vi "xy_graph_zoom.vi"() -> ()   [LabVIEW 2009]
uses:
  <vilib>/Utility/file.llb/Write To Spreadsheet File (DBL).vi
panel:
  out "sub-array for csv file":dbl[][](array[numeric])
  in  "stop":bool
  out "csv":bool
  out "print":bool
  in  "csv":bool
  in  "print":bool
  out "y-axis of sub-array":dbl[](array[numeric])
  out "x-axis of sub-array":dbl[](array[numeric])
  out "Y-max":dbl
  out "Y-min":dbl
  out "X-max":dbl
  out "X-min":dbl
  in  "y-axis array":dbl[](array[numeric])=[6.0, 2.0, 3.0, 9.0, 8.0, 5.0, 12.0, 14.0, 7.0, 18.0, 16.0]
  in  "x-axis array":dbl[](array[numeric])=[0.0, 2.0, 4.0, 6.0, 8.0, 10.0, 12.0, 14.0, 16.0, 18.0, 20.0]
  out "XY Graph":cluster{"Array":dbl[], "Array 2":dbl[]}(graph)
  # "these will write to C:\\temp\\ (the directory must exist)"
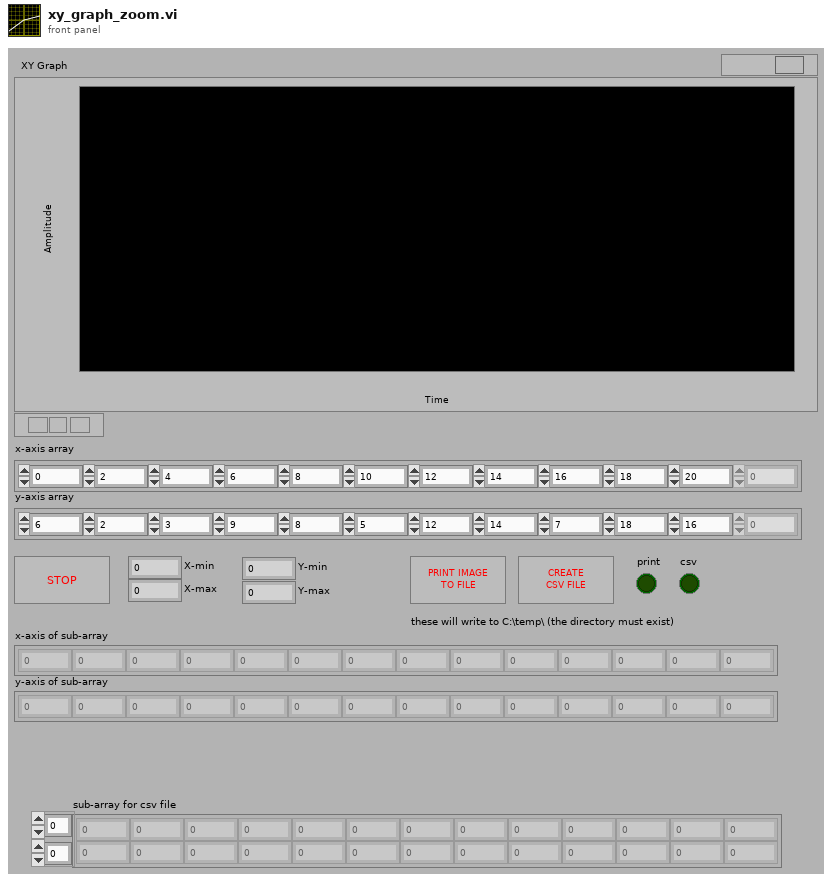
[diagram p1: front panel]
types:
  T1 = cluster{"x-axis array":dbl[], "y-axis array":dbl[]}
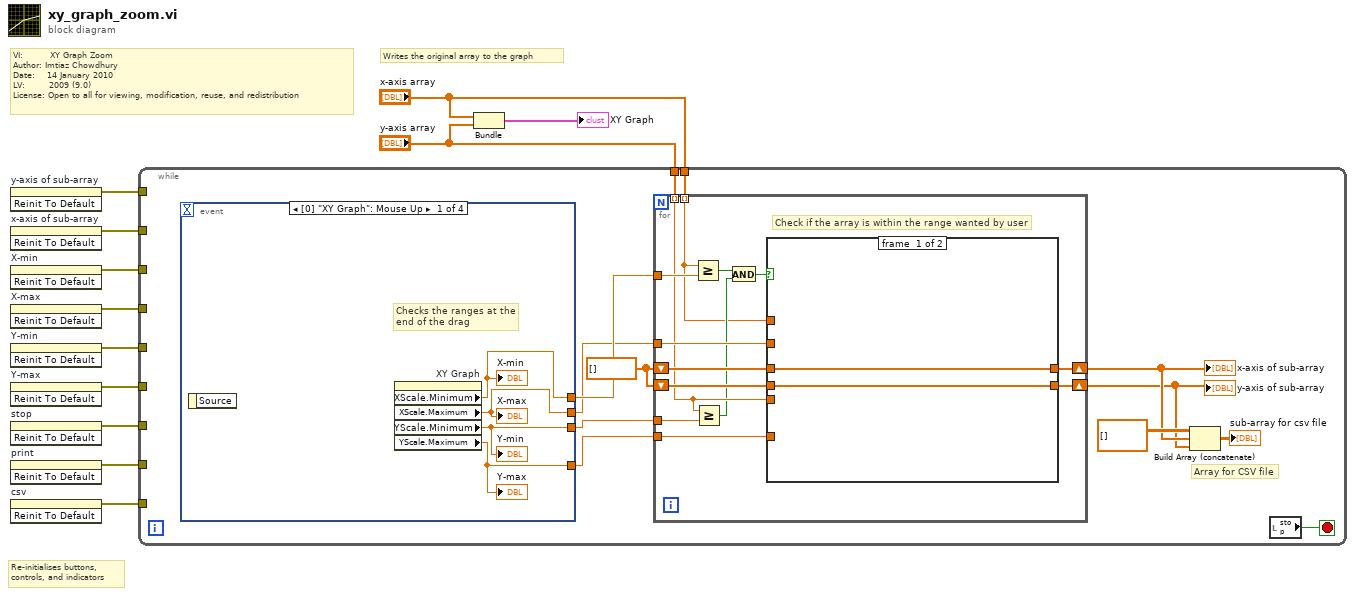
[diagram p0: block diagram]
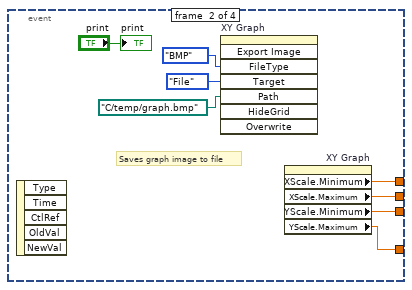
[diagram p2: hidden frame]
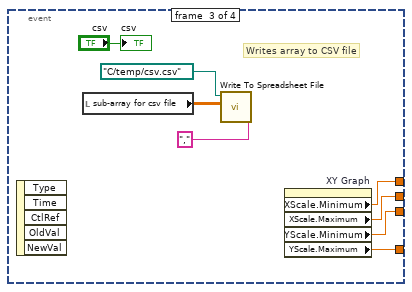
[diagram p3: hidden frame]
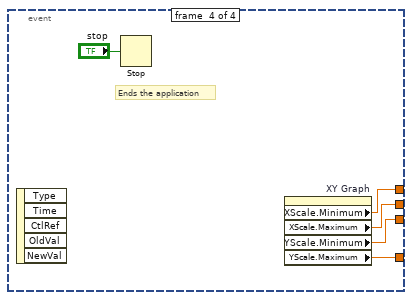
[diagram p4: hidden frame]
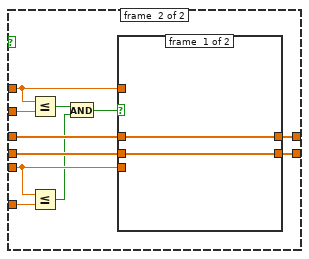
[diagram p5: hidden frame]
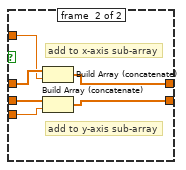
[diagram p6: hidden frame]
diagram:
  # "VI:         XY Graph Zoom\nAuthor: Imtiaz Chowdhury\nDate:    14 January 2010\nLV:        2009 (9.0)\nLicense: Open to all for viewing, modification, reuse, and redistribution"
  # "Writes the original array to the graph"
  # "Re-initialises buttons,\ncontrols, and indicators"
  n1 = invoke on="y-axis of sub-array" class="Arr (strict)" method="Reinit To Default"() -> (error out=w3:errorcluster)  [unwired: 3 in, 2 out]
  n2 = invoke on="x-axis of sub-array" class="Arr (strict)" method="Reinit To Default"() -> (error out=w4:errorcluster)  [unwired: 3 in, 2 out]
  n3 = invoke on="X-min" class="DigNum (strict)" method="Reinit To Default"() -> (error out=w5:errorcluster)  [unwired: 3 in, 2 out]
  n4 = invoke on="X-max" class="DigNum (strict)" method="Reinit To Default"() -> (error out=w6:errorcluster)  [unwired: 3 in, 2 out]
  n5 = invoke on="Y-min" class="DigNum (strict)" method="Reinit To Default"() -> (error out=w7:errorcluster)  [unwired: 3 in, 2 out]
  n6 = invoke on="Y-max" class="DigNum (strict)" method="Reinit To Default"() -> (error out=w8:errorcluster)  [unwired: 3 in, 2 out]
  n7 = invoke on="stop" class="Bool (strict)" method="Reinit To Default"() -> (error out=w9:errorcluster)  [unwired: 3 in, 2 out]
  n8 = invoke on="print" class="Bool (strict)" method="Reinit To Default"() -> (error out=w10:errorcluster)  [unwired: 3 in, 2 out]
  n9 = invoke on="csv" class="Bool (strict)" method="Reinit To Default"() -> (error out=w11:errorcluster)  [unwired: 3 in, 2 out]
  n10 = while {
    tunnel: w11 -> [_]
    tunnel: w10 -> [_]
    tunnel: w9 -> [_]
    tunnel: w8 -> [_]
    tunnel: w7 -> [_]
    tunnel: w6 -> [_]
    tunnel: w5 -> [_]
    tunnel: w4 -> [_]
    tunnel: w3 -> [_]
    tunnel: "y-axis array" -> [w14]
    tunnel: "x-axis array" -> [w13]
    stop <- w23 stop-if-true
    w24 = dbl[] [] ("Array 3")
    # "Array for CSV file"
    n11 = event shown="[0] \"XY Graph\": Mouse Up" {
      selector: _ -> [_ _ _ _]
      dyn-events: _ -> [_ _ _ _]
      timeout: _ -> [_ _ _ _]
      tunnel: [w28 w35 w38 w48] -> w22
      tunnel: [w27 w31 w40 w47] -> w17
      tunnel: [w26 w30 w39 w46] -> w16
      tunnel: [w25 w29 w37 w45] -> w15
      event #0 {
        # "Checks the ranges at the\nend of the drag"
        n12 = event-data() -> ()  [unwired: 1 in, 1 out]
        n13 = property on="XY Graph" class="XYGraph (strict)"() -> ("XScale.Minimum"=w27:dbl, "XScale.Maximum"=w26:dbl, "YScale.Minimum"=w28:dbl, "YScale.Maximum"=w25:dbl)  [unwired: 2 in, 2 out]
        "X-min" <- w27
        "X-max" <- w26
        "Y-min" <- w28
        "Y-max" <- w25
      }
      event #1 {
        # "Saves graph image to file"
        n14 = event-data() -> ()  [unwired: 1 in, 5 out]
        n15 = invoke on="XY Graph" class="XYGraph (strict)" method="Export Image"("FileType"=enum32{"BMP", "EPS", "EMF", "PICT"}."BMP" ("File Type"), "Target"=enum32{"File", "Clipboard"}."File", "Path"=path "C:/temp/graph.bmp") -> ()  [unwired: 5 in, 8 out]
        n16 = property on="XY Graph" class="XYGraph (strict)"() -> ("XScale.Minimum"=w31:dbl, "XScale.Maximum"=w30:dbl, "YScale.Minimum"=w35:dbl, "YScale.Maximum"=w29:dbl)  [unwired: 2 in, 2 out]
        "print" <- "print"
      }
      event #2 {
        # "Writes array to CSV file"
        n17 = event-data() -> ()  [unwired: 1 in, 5 out]
        n18 = local read "sub-array for csv file"() -> (w42:dbl[][])
        n19 = call-poly <vilib>:"Write To Spreadsheet File.vi"("delimiter (\\t)"="," ("delimiter (\\t)"), "2D data"=w42, "file path (dialog if empty)"=path "C:/temp/csv.csv") -> ()  [unwired: 5 in, 1 out]
        n20 = property on="XY Graph" class="XYGraph (strict)"() -> ("XScale.Minimum"=w40:dbl, "XScale.Maximum"=w39:dbl, "YScale.Minimum"=w38:dbl, "YScale.Maximum"=w37:dbl)  [unwired: 2 in, 2 out]
        "csv" <- "csv"
      }
      event #3 {
        # "Ends the application"
        n21 = event-data() -> ()  [unwired: 1 in, 5 out]
        n22 = Stop(stop? (T)="stop") -> ()
        n23 = property on="XY Graph" class="XYGraph (strict)"() -> ("XScale.Minimum"=w47:dbl, "XScale.Maximum"=w46:dbl, "YScale.Minimum"=w48:dbl, "YScale.Maximum"=w45:dbl)  [unwired: 2 in, 2 out]
      }
    }
    n24 = for {
      tunnel: w13 -> [w51] mode=indexing
      tunnel: w17 -> [w62]
      tunnel: w16 -> [w61]
      shift-right: [w59] -> w20
      shift-left: w24 -> [w60]
      shift-right: [w57] -> w19
      shift-left: w24 -> [w58]
      tunnel: w14 -> [w56] mode=indexing
      tunnel: w22 -> [w55]
      tunnel: w15 -> [w50]
      # "Check if the array is within the range wanted by user"
      n25 = Greater Or Equal?(x=w51, y=w62) -> (x >= y?=w54:bool)
      n26 = Greater Or Equal?(x=w56, y=w55) -> (x >= y?=w52:bool)
      n27 = And(x=w54, y=w52) -> (x .and. y?=w53:bool)
      n28 = case shown="True" w53 {
        tunnel: w61 -> [_ w75]
        tunnel: w60 -> [w64 w74]
        tunnel: [w64 w73] -> w59
        tunnel: w58 -> [w63 w72]
        tunnel: [w63 w71] -> w57
        tunnel: w56 -> [_ w70]
        tunnel: w51 -> [_ w66]
        tunnel: w50 -> [_ w65]
        frame #0 {
        }
        frame #1 {
          n29 = Less Or Equal?(x=w66, y=w75) -> (x <= y?=w69:bool)
          n30 = Less Or Equal?(x=w70, y=w65) -> (x <= y?=w67:bool)
          n31 = And(x=w69, y=w67) -> (x .and. y?=w68:bool)
          n32 = case shown="True" w68 {
            tunnel: w66 -> [_ w82]
            tunnel: w74 -> [w77 w83]
            tunnel: [w77 w81] -> w73
            tunnel: w72 -> [w76 w80]
            tunnel: [w76 w79] -> w71
            tunnel: w70 -> [_ w78]
            frame #0 {
            }
            frame #1 {
              # "add to y-axis sub-array"
              # "add to x-axis sub-array"
              n33 = Build Array (concatenate)(w83, w82) -> (w81:dbl[])
              n34 = Build Array (concatenate)(w80, w78) -> (w79:dbl[])
            }
          }
        }
      }
    }
    "x-axis of sub-array" <- w20
    "y-axis of sub-array" <- w19
    n35 = Build Array (concatenate)(dbl[][] [] ("Array 3"), w20, w19) -> (→"sub-array for csv file":dbl[][])
    n36 = local read "stop"() -> (w23:bool)
  }
  n37 = Bundle("x-axis array"="x-axis array", "y-axis array"="y-axis array") -> (→"XY Graph":T1)  [unwired: 1 in]
